vi "test Secure Client.vi"(8 "error in (no error)":errorcluster, 11 "TestCase in":refnum<class "test Secure Socket.lvclass">) -> (0 "error out":errorcluster, 3 "TestCase out":refnum<class "test Secure Socket.lvclass">)   [LabVIEW 2013, in "test Secure Socket.lvclass"]
uses:
  test Secure Socket.lvclass
  SSL_Lib/SSL-Context/SSL Verify Mode.ctl
  SSL_Lib/SSL-Context/SSL Options.ctl
  SSL_Lib/SSL-Lib/Library Paths.ctl
  SSL Client Context/SSL Client Context.lvclass/SSL Client Context.ctl
  SSL Client Context/SSL Client Context.lvclass
  SSL Client Socket/SSL Client Socket.lvclass
  SSL Client Context/Write Verification Options.vi
  SSL Client Context/Write Verification CA Bundle Path.vi
  SSL Client Context/Write SSL Options.vi
  SSL Client Context/Write Cipher List.vi
  <vilib>/addons/_JKI Toolkits/VI Tester/TestCase.llb/TestCase.lvclass
  SSL_Lib/SSL-Context/SSL-Context.lvclass
  SSL_Lib/SSL-Lib/SSL-Lib.lvclass
panel:
  out "bytes written":i32
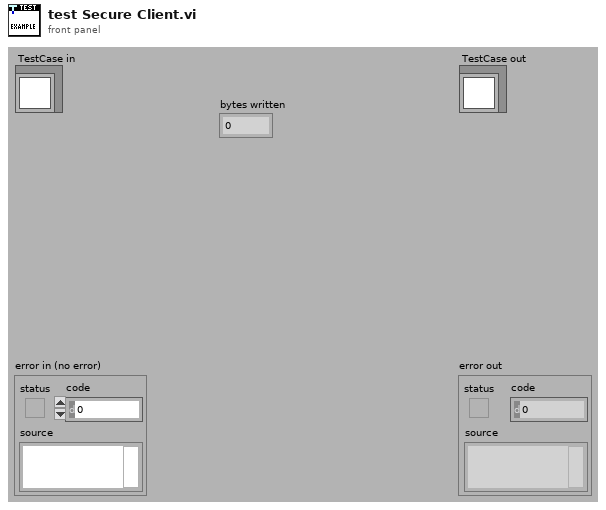
[diagram p1: front panel]
types:
  T1 = typedef "SSL_Lib.lvlib/SSL-Lib.lvclass/Library Paths.ctl" = cluster{"SSL Library Path":path, "Crypto Library Path":path}
  T2 = typedef "SSL_Lib.lvlib/SSL-Context.lvclass/SSL Options.ctl" = i32
  T3 = typedef "SSL_Lib.lvlib/SSL-Context.lvclass/SSL Verify Mode.ctl" = i32
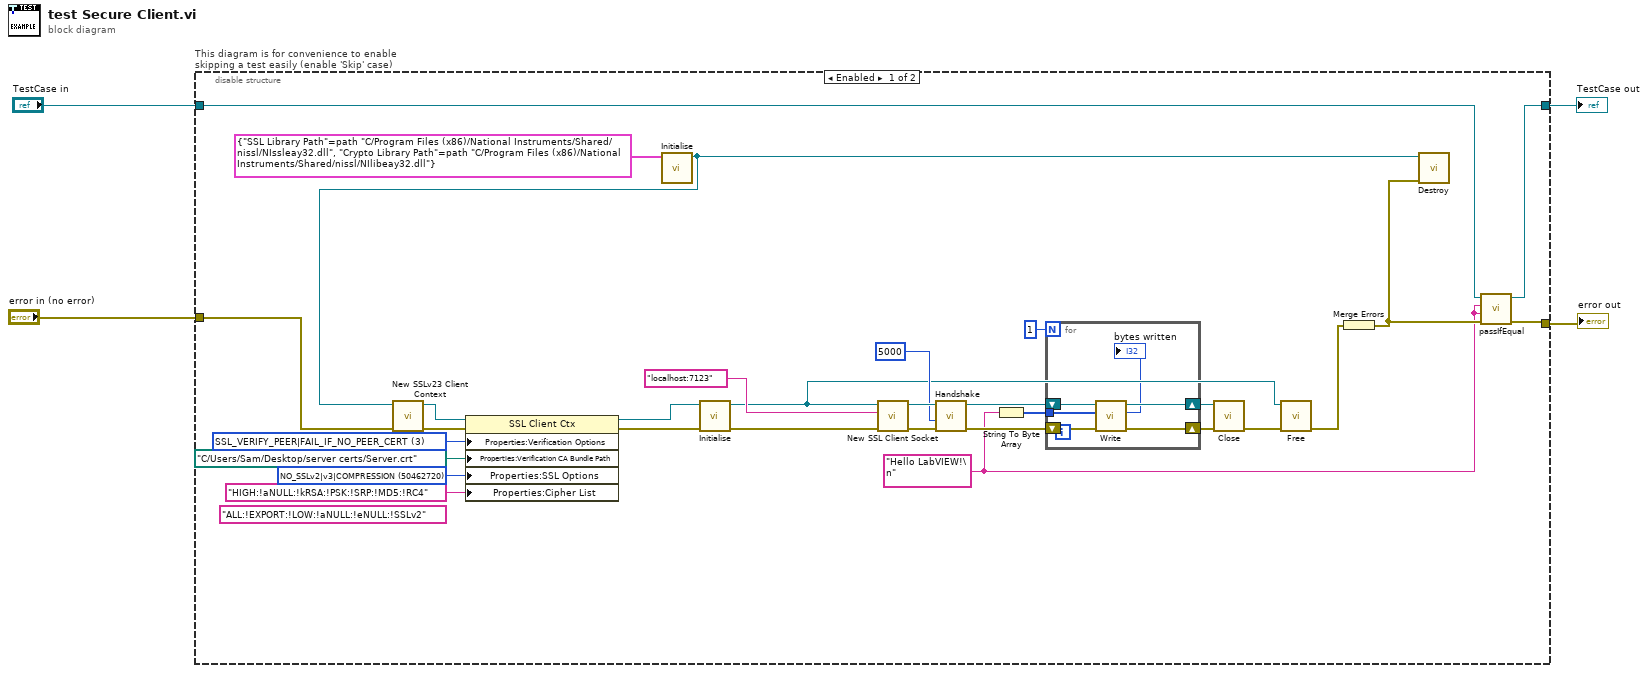
[diagram p0: block diagram]
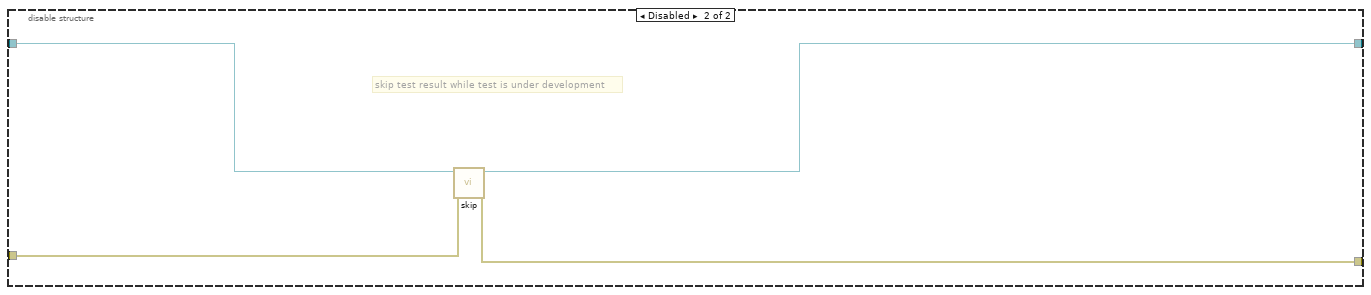
[diagram p2: hidden frame]
diagram:
  n1 = disable-structure "This diagram is for convenience to enable skipping a test easily (enable 'Skip' case)" shown="Enabled" {
    disable-tunnel: "TestCase in" -> [w32 w44]
    disable-tunnel: [w34 w42] -> w1
    disable-tunnel: [w33 w43] -> w3
    disable-tunnel: "error in (no error)" -> [w24 w41]
    frame Enabled {
      w6 = "Hello LabVIEW!\n"
      (unwired) "ALL:!EXPORT:!LOW:!aNULL:!eNULL:!SSLv2" ("Cipher List")
      w25 = T2 50462720 items=["None"=0, "NO_SSLv2|v3|COMPRESSION"=50462720, "SSL_OP_NO_COMPRESSION"=131072, "SSL_OP_NO_SSLv2"=16777216, "SSL_OP_NO_SSLv3"=33554432, "SSL_OP_NO_TLSv1"=67108864, "SSL_OP_NO_TLSv1_2"=134217728, "SSL_OP_NO_TLSv1_1"=268435456] ("SSL Options")
      w27 = T3 3 items=["SSL_VERIFY_PEER|FAIL_IF_NO_PEER_CERT"=3, "SSL_VERIFY_NONE"=0, "SSL_VERIFY_PEER"=1, "SSL_VERIFY_FAIL_IF_NO_PEER_CERT"=2, "SSL_VERIFY_CLIENT_ONCE"=4] ("Verification Options")
      n2 = call "Initialise.vi"("Library Paths"=T1 {"SSL Library Path"=path "C:/Program Files (x86)/National Instruments/Shared/nissl/NIssleay32.dll", "Crypto Library Path"=path "C:/Program Files (x86)/National Instruments/Shared/nissl/NIlibeay32.dll"}) -> ("SSL-Lib out"=w8:refnum<class "SSL-Lib.lvclass">)  [unwired: 9 in, 1 out]
      n3 = call "New SSLv23 Client Context.vi"("error in (no error)"=w24, "SSL-Lib"=w8) -> ("error out"=w31:errorcluster, "SSL Client Context out"=w29:refnum<class "SSL Client Context.lvclass">)  [unwired: 8 in]
      n4 = property class="SSL Client Ctx"(reference=w29, error in=w31, "Properties:Verification Options"=w27, "Properties:Verification CA Bundle Path"=path "C:/Users/Sam/Desktop/server certs/Server.crt" ("Path to CA bundle"), "Properties:SSL Options"=w25, "Properties:Cipher List"="HIGH:!aNULL:!kRSA:!PSK:!SRP:!MD5:!RC4" ("Cipher List")) -> (reference out=w28:refnum<class "SSL Client Context.lvclass">, error out=w30:errorcluster)
      n5 = call-dynamic "Initialise.vi"("error in (no error)"=w30, "OpenSSL Client Context in"=w28) -> ("error out"=w20:errorcluster, "OpenSSL Client Context out"=w10:refnum<class "SSL Client Context.lvclass">)  [unwired: 8 in]
      n6 = call "New SSL Client Socket.vi"("error in (no error)"=w20, "Hostname / URL"="localhost:7123", "SSL Client Ctx"=w10) -> ("error out"=w21:errorcluster, "SSL Client Skt out"=w22:refnum<class "SSL Client Socket.lvclass">)  [unwired: 7 in]
      n7 = call-dynamic "Handshake.vi"("error in (no error)"=w21, "Timeout (5000ms)"=u32 5000, "OpenSSL in"=w22) -> ("error out"=w17:errorcluster, "OpenSSL out"=w16:refnum<class "SSL Client Socket.lvclass">)  [unwired: 7 in]
      n8 = String To Byte Array(string=w6) -> (unsigned byte array=w14:u8[])
      n9 = for {
        N: 1 -> [_]
        tunnel: w14 -> [w37]
        shift-right: [w38] -> w15
        shift-left: w16 -> [w39]
        shift-right: [w36] -> w13
        shift-left: w17 -> [w40]
        n10 = call-dynamic "Write.vi"("error in (no error)"=w40, "Bytes to write"=w37, "OpenSSL Socket in"=w39) -> ("error out"=w36:errorcluster, "bytes written"=→"bytes written":i32, "OpenSSL Socket out"=w38:refnum<class "SSL Client Socket.lvclass">)  [unwired: 6 in]
      }
      n11 = call-dynamic "Close.vi"("error in (no error)"=w13, "OpenSSL Socket in"=w15) -> ("error out"=w12:errorcluster)  [unwired: 9 in]
      n12 = call-dynamic "Free.vi"("error in (no error)"=w12, "OpenSSL Context in"=w10) -> ("error out"=w11:errorcluster)  [unwired: 9 in]
      n13 = Merge Errors(w11) -> (w7:errorcluster)
      n14 = call "Destroy.vi"("error in (no error)"=w7, "SSL-Lib in"=w8) -> ()  [unwired: 9 in, 1 out]
      n15 = call-dynamic "passIfEqual.vi"("error in (no error)"=w7, "y"=w6, "x"=w6, "TestCase in"=w32) -> ("error out"=w33:errorcluster, "TestCase out"=w34:refnum<class "test Secure Socket.lvclass">)  [unwired: 6 in]
    }
    frame Disabled {
      # "skip test result while test is under development"
      n16 = call <vilib>:"skip.vi"("error in (no error)"=w41, "TestCase in"=w44) -> ("error out"=w43:errorcluster, "TestCase out"=w42:refnum<class "test Secure Socket.lvclass">)  [unwired: 8 in]
    }
  }
  "error out" <- w3
  "TestCase out" <- w1
